vi "Dryer.vi"() -> ()   [LabVIEW 2019]
uses:
  <vilib>/NI/Current Value Table/Type Defs/Single Tag.ctl
  <vilib>/NI/Current Value Table/Type Defs/Data Types.ctl
  <vilib>/NI/STM/TCP/Read Meta Data (TCP Ref).vi
  <vilib>/NI/STM/TCP/Get Connection Reference (TCP).vi
  <vilib>/NI/AMC/Read Termination Message.vi
  <vilib>/NI/AMC/Create Single Message.vi
  <vilib>/NI/AMC/Update Message Routing Info.vi
  <vilib>/NI/STM/TCP/Read Meta Data (TCP Clst).vi
  <vilib>/NI/AMC/Globals.vi
  <vilib>/NI/STM/TCP/Write Message (TCP).vi
  <vilib>/NI/AMC/Send Message.vi
  <vilib>/NI/AMC/AMC.lvlib
  <vilib>/NI/STM/NI STM.lvlib
  <vilib>/NI/Current Value Table/Current Value Table.lvlib
panel:
  in  "Drying Flow %":dbl(knob)=5.0 min=5.0 max=50.0 step=0.1 scale=0.0..100.0
  in  "Standby Flow %":dbl(knob)=5.0 min=5.0 max=50.0 step=0.1 scale=0.0..100.0
  in  "PlenumWtrT Last Hr":bool
  out "Plenum Water Exit T":dbl(slide) scale=0.0..100.0
  in  "DryerBlrVlv Last Hr":bool
  in  "DryerT Last Hr":bool
  out "Boiler Water Valve Position":dbl(knob) scale=0.0..100.0
  out "E Stop":bool
  out "Run Enabled?":bool
  out "Actual Temperature":dbl(knob) scale=0.0..100.0
  in  "Temperature Setpoint":dbl(knob)=20.0 min=20.0 max=70.0 step=1.0 scale=20.0..70.0
  in  "Enable Dryer":bool
  in  "Machine":bool
  in  "Basement 4":bool
  in  "Dryer":bool
  in  "Rinse 4":bool
  in  "Rinse 3":bool
  in  "Rinse 2":bool
  in  "Basement 3":bool
  in  "Basement 2":bool
  in  "Basement 1":bool
  in  "Plater 6":bool
  in  "Plater 5":bool
  in  "Plater 4":bool
  in  "Plater 3":bool
  in  "Plater 2":bool
  in  "Plater 1":bool
  in  "Predip":bool
  in  "Rinse 1":bool
  in  "Cleaner":bool
  in  "Etch":bool
  out "status":string
  # "Module Selection"
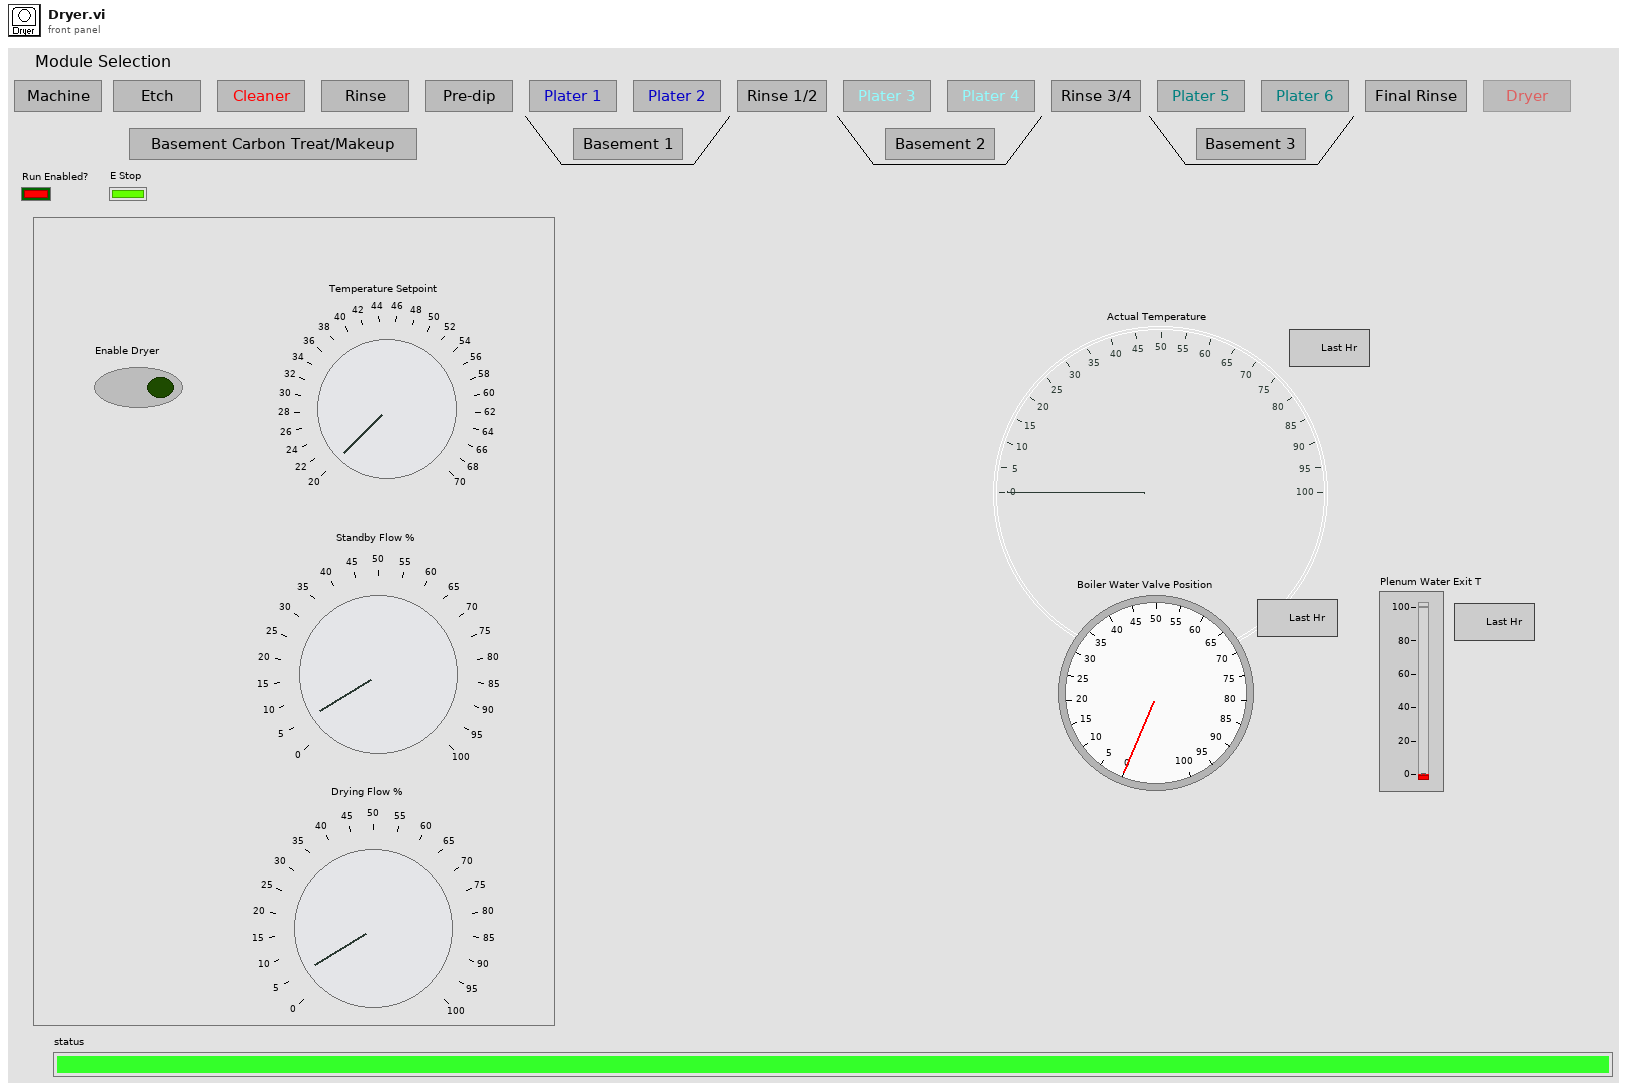
[diagram p1: front panel]
types:
  T1 = typedef "Current Value Table.lvlib/Single Tag.ctl" = cluster{"Data Type":T2, "Name":string, "Value":string, "Description":string}
  T2 = typedef "Current Value Table.lvlib/Data Types.ctl" = enum16{"Double", "Single", "I64", "I32", "I16", "I8", "U64", "U32", "U16", "U8", "String", "Boolean", "Array of U8", "Array of U16", "Array of U32", "Array of U64", "Array of I64", "Array of I32", "Array of I16", "Array of I8", "Array of Double", "Array of Single", "Array of Boolean", "Array of String"}
  T3 = typedef "NI STM.lvlib/TCP Connection Info.ctl" = cluster{"connection ID":refnum<k5>, "meta data":T4[]}
  T4 = typedef "NI STM.lvlib/MetaDataElement.ctl" = string
  T5 = typedef "AMC.lvlib/Message Queue.ctl" = refnum<queue>
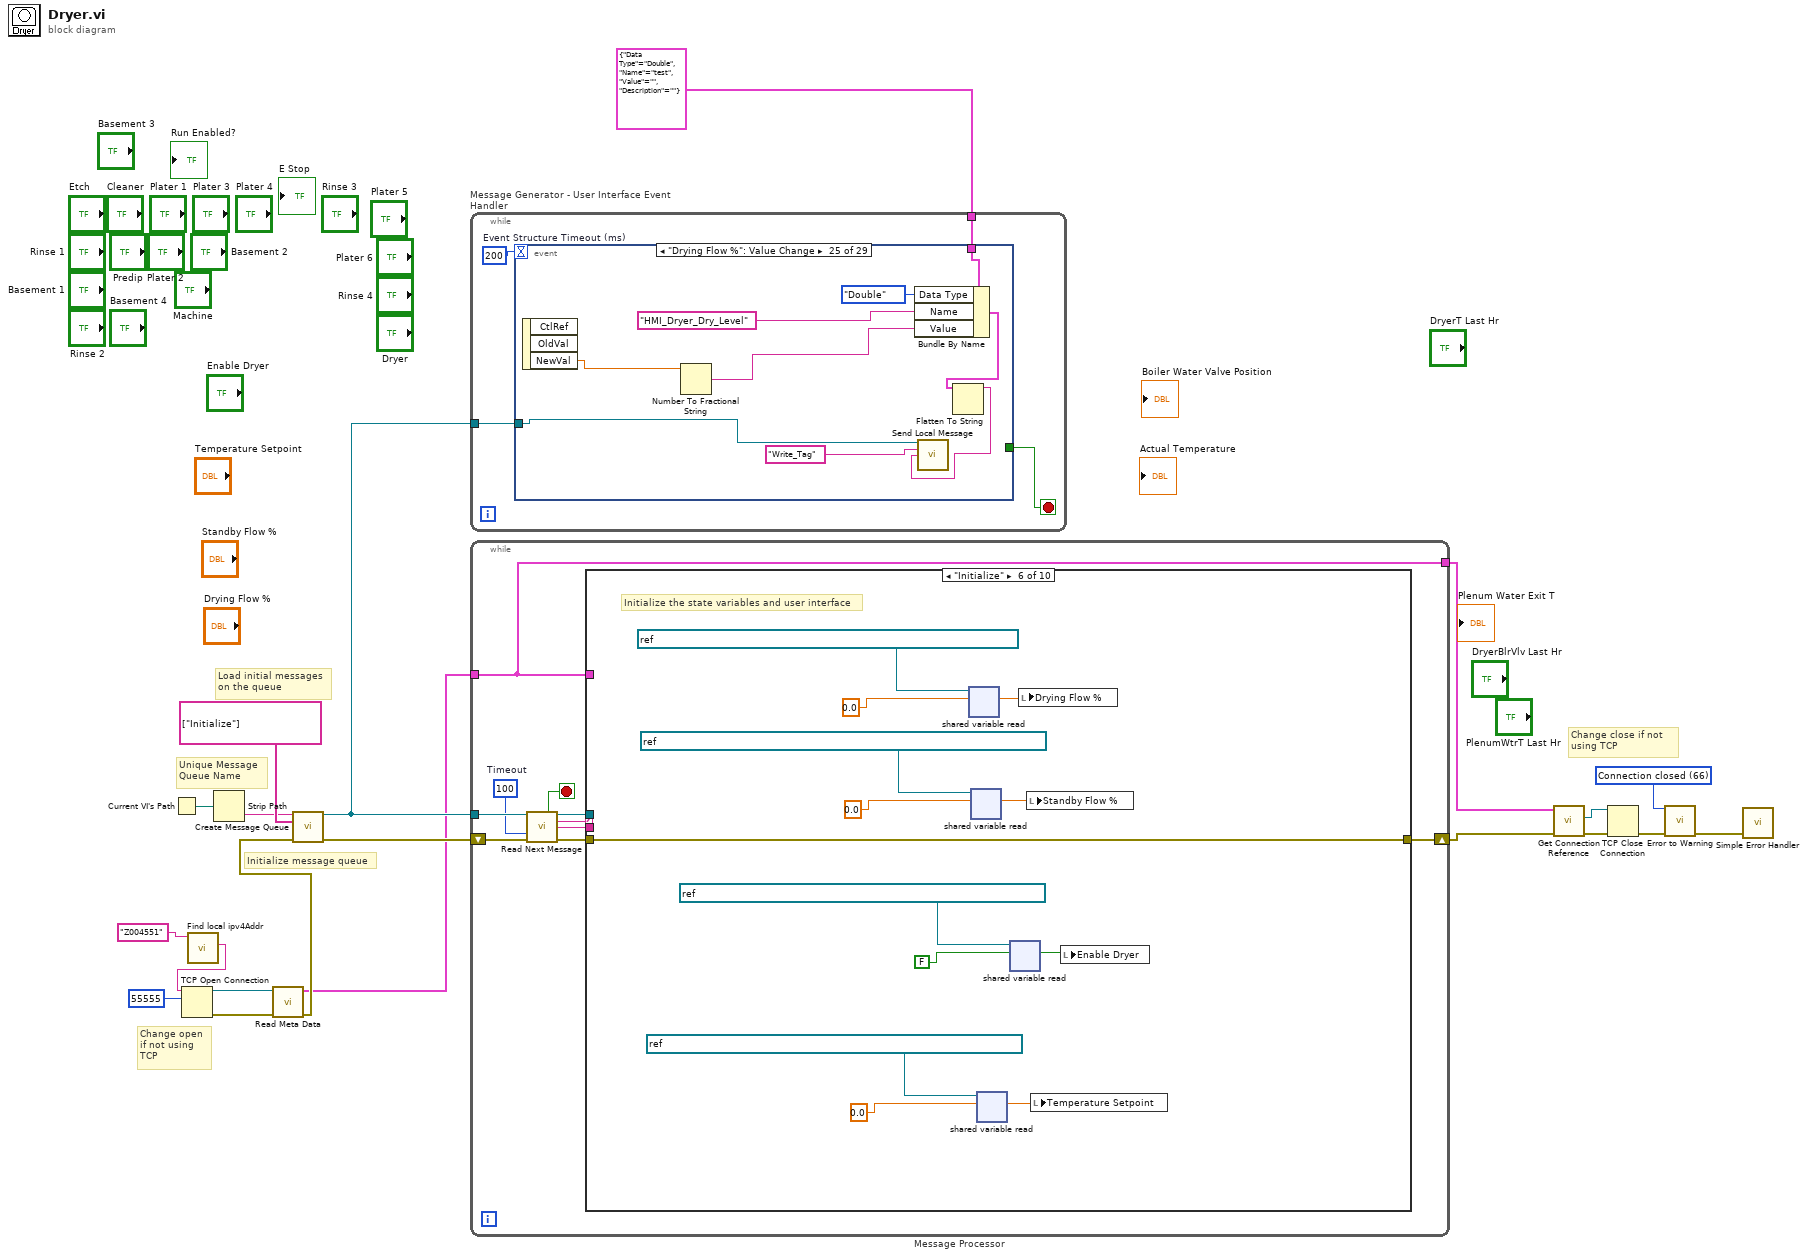
[diagram p0: block diagram]
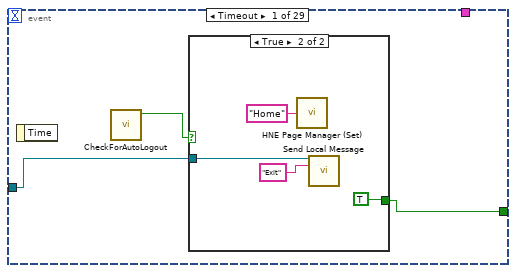
[diagram p2: hidden frame]
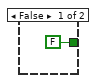
[diagram p3: hidden frame]
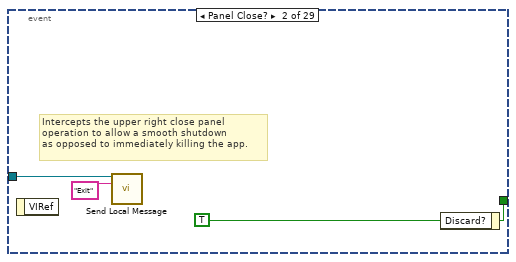
[diagram p4: hidden frame]
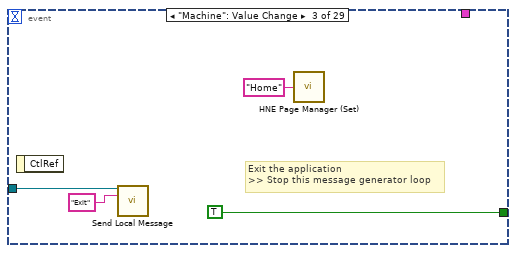
[diagram p5: hidden frame]
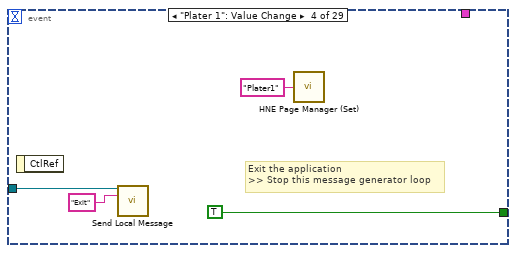
[diagram p6: hidden frame]
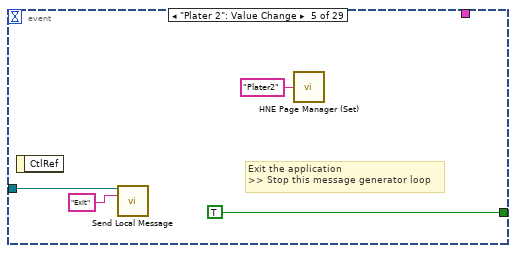
[diagram p7: hidden frame]
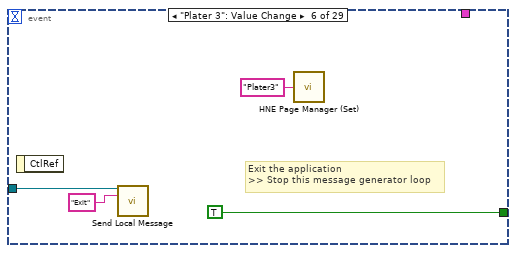
[diagram p8: hidden frame]
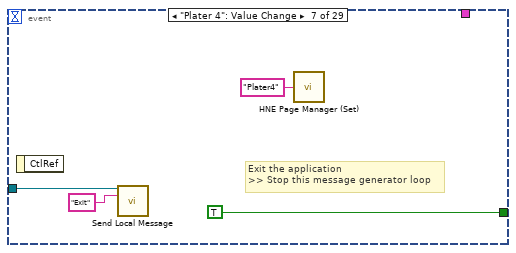
[diagram p9: hidden frame]
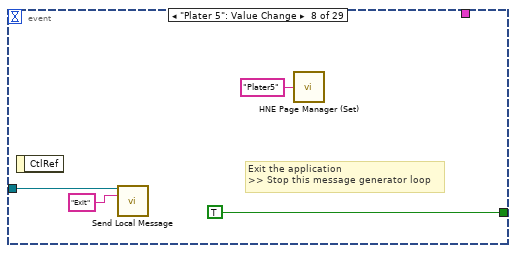
[diagram p10: hidden frame]
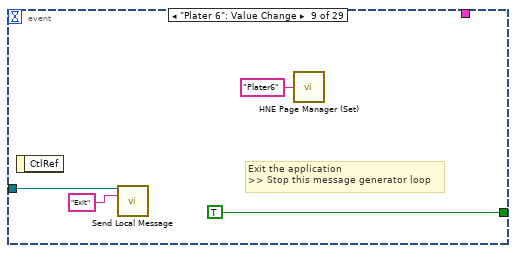
[diagram p11: hidden frame]
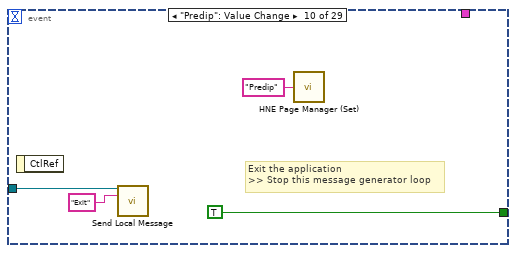
[diagram p12: hidden frame]
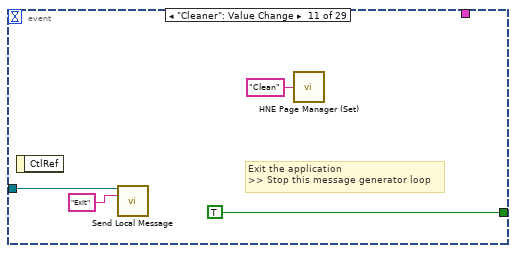
[diagram p13: hidden frame]
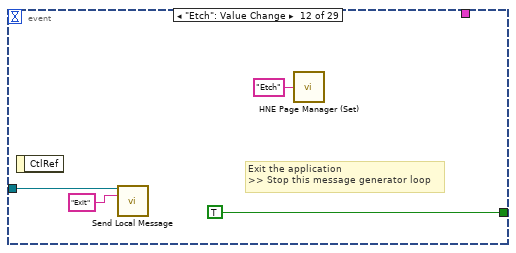
[diagram p14: hidden frame]
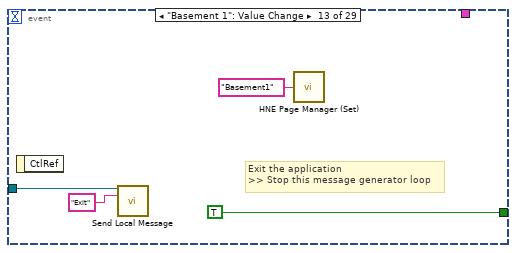
[diagram p15: hidden frame]
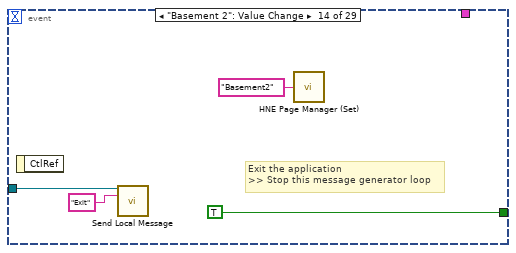
[diagram p16: hidden frame]
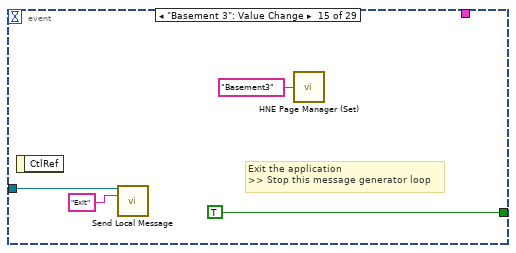
[diagram p17: hidden frame]
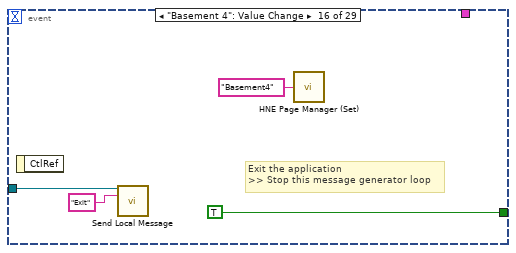
[diagram p18: hidden frame]
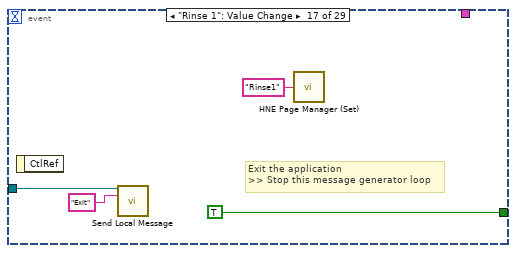
[diagram p19: hidden frame]
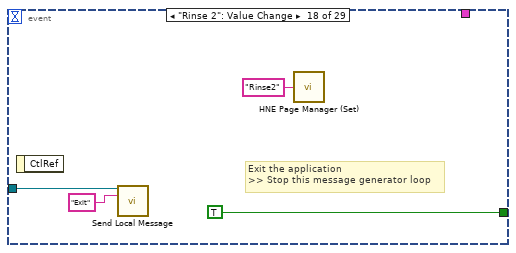
[diagram p20: hidden frame]
diagram:
  w9 = 66 items=["No Error", "Argument Error", "Memory Full", "Out of Zone", "End of File", "File Already Open", "Generic File IO Error", "File Not Found", "File Permission Error", "Disk Full", "Duplicate Path", "Too Many Files Open", "Not Enabled", "Resource File Not Found", "Cannot Add Resource", "Resource Not Found", "Image Not Found", "Image Memory Error", "Pen Does Not Exist", "Config Bad Type", "Config Token Not Found", "Config Parse Error", "Config Memory Error", "Bad External Code Format", "Bad External Code Offset", "External Code Not Present", "Null Window", "Destroy Window Mixup", "Null Menu", "Print Aborted", "Bad Print Record", "Print Driver Error", "Windows Error During Print", "Memory Error During Print", "Print Dialog Error", "Generic Print Error", "Invalid Device Refnum", "Device Not Found", "Device Parameter Error", "Device Unit Error", "Can't Open Device", "Device Call Aborted", "Generic Error", "Cancelled By User", "Object ID Too Low", "Object ID Too High", "Object Not In Heap", "Unknown Heap", "Bad DefProc ID", "DefProc Not In Table", "Message Out Of Range", "Null Method", "Unknown Message", "Manager Call Not Supported", "Bad address", "Connection In progress", "Connection timed out", "Connection is already in progress", "Network attribute not supported", "Network error", "Address in use", "System out of memory", "Connection aborted", "Connection refused", "Connection is not connected", "Connection is already connected", "Connection closed", "Initialize error (interapplication manager)", "Bad occurrence", "Wait on unbound occurrence handler", "Occurrence queue overflow", "Bad path", "Semaphore not signaled", "Unrecognized type (interapplication manager)"] ("1st Error to Convert")
  # "Change close if not using TCP"
  # "Change open if not using TCP"
  # "Initialize message queue"
  # "Unique Message\nQueue Name"
  # "Load initial messages\non the queue"
  n1 = Current VI's Path() -> (path=w16:path)
  n2 = call "Find local ipv4Addr.vi"("MachineToFind"="Z004551" ("Target IP Address")) -> ("name"=w2:string)  [unwired: 9 in, 1 out]
  n3 = TCP Open Connection(address=w2, remote port or service name=u16 55555 ("remote port")) -> (connection ID=w14:refnum<k5>, error out=w13:errorcluster)  [unwired: 1 in, 2 out]
  n4 = Strip Path(path=w16) -> (name=w19:string)  [unwired: 1 out]
  n5 = call-poly <vilib>:"Read Meta Data.vi"("error in"=w13, "connection ID"=w14) -> ("error out"=w12:errorcluster, "connection info out"=w11:T3)  [unwired: 7 in, 1 out]
  n6 = call <vilib>:"Create Message Queue.vi"("message queue name"=w19, "initial message names"=string[] ["Initialize"], "error in"=w12) -> ("message queue out"=w18:T5, "error out"=w17:errorcluster)  [unwired: 11 in]
  n7 = while "Message Generator - User Interface Event Handler" {
    tunnel: w18 -> [w22]
    tunnel: T1 {"Data Type"=enum."Double", "Name"="test", "Value"="", "Description"=""} ("Tag") -> [w21]
    stop <- w23 stop-if-true
    w24 = 200  # Event Structure Timeout (ms)
    n8 = event shown="[24] \"Drying Flow %\": Value Change" {
      selector: _ -> [_ _ _ _ _ _ _ _ _ _ _ _ _ _ _ _ _ _ _ _ _ _ _ _ _ _ _ _ _]
      dyn-events: _ -> [_ _ _ _ _ _ _ _ _ _ _ _ _ _ _ _ _ _ _ _ _ _ _ _ _ _ _ _ _]
      timeout: w24 -> [_ _ _ _ _ _ _ _ _ _ _ _ _ _ _ _ _ _ _ _ _ _ _ _ _ _ _ _ _]
      tunnel: [w25 w35 TRUE ("Discard?") TRUE ("Discard?") TRUE ("Discard?") TRUE ("Discard?") TRUE ("Discard?") TRUE ("Discard?") TRUE ("Discard?") TRUE ("Discard?") TRUE ("Discard?") TRUE ("Discard?") TRUE ("Discard?") TRUE ("Discard?") TRUE ("Discard?") TRUE ("Discard?") TRUE ("Discard?") TRUE ("Discard?") TRUE ("Discard?") TRUE ("Discard?") TRUE ("Discard?") _ _ _ _ _ _ _ _] -> w23
      tunnel: w22 -> [w26 w33 w37 w41 w45 w49 w53 w57 w61 w65 w69 w73 w77 w81 w85 w89 w93 w97 w101 w105 w109 w115 w126 w135 w144 w149 w154 w159 w164]
      tunnel: w21 -> [_ _ _ _ _ _ _ _ _ _ _ _ _ _ _ _ _ _ _ _ _ w113 w125 w134 w143 _ _ _ _]
      event Timeout {
        n9 = event-data() -> ()  [unwired: 2 out]
        n10 = call "CheckForAutoLogout.vi"() -> ("Boolean"=w27:bool)  [unwired: 11 in]
        n11 = case shown="True" w27 {
          tunnel: [FALSE ("Discard?") TRUE ("Discard?")] -> w25
          tunnel: w26 -> [_ w29]
          frame False {
          }
          frame True {
            n12 = call <userlib>:"HNE Page Manager (Set).vi"("Next Page"="Home") -> ()  [unwired: 4 in, 1 out]
            n13 = call <vilib>:"Send Local Message.vi"("message queue in"=w29, "message name"="Exit") -> ()  [unwired: 11 in, 3 out]
          }
        }
      }
      event Panel Close? {
        w35 = TRUE ("Discard?")
        # "Intercepts the upper right close panel\noperation to allow a smooth shutdown\nas opposed to immediately killing the app."
        n14 = event-data() -> ()  [unwired: 2 out]
        n15 = call <vilib>:"Send Local Message.vi"("message queue in"=w33, "message name"="Exit") -> ()  [unwired: 11 in, 3 out]
        n16 = event-data("Discard?"=w35) -> ()  [unwired: 1 in, 1 out]
      }
      event "Machine": Value Change {
        # "Exit the application\n>> Stop this message generator loop"
        n17 = event-data() -> ()  [unwired: 2 out]
        n18 = call <vilib>:"Send Local Message.vi"("message queue in"=w37, "message name"="Exit") -> ()  [unwired: 11 in, 3 out]
        n19 = call <userlib>:"HNE Page Manager (Set).vi"("Next Page"="Home") -> ()  [unwired: 4 in, 1 out]
      }
      event "Plater 1": Value Change {
        # "Exit the application\n>> Stop this message generator loop"
        n20 = event-data() -> ()  [unwired: 2 out]
        n21 = call <vilib>:"Send Local Message.vi"("message queue in"=w41, "message name"="Exit") -> ()  [unwired: 11 in, 3 out]
        n22 = call <userlib>:"HNE Page Manager (Set).vi"("Next Page"="Plater1") -> ()  [unwired: 4 in, 1 out]
      }
      event "Plater 2": Value Change {
        # "Exit the application\n>> Stop this message generator loop"
        n23 = event-data() -> ()  [unwired: 2 out]
        n24 = call <vilib>:"Send Local Message.vi"("message queue in"=w45, "message name"="Exit") -> ()  [unwired: 11 in, 3 out]
        n25 = call <userlib>:"HNE Page Manager (Set).vi"("Next Page"="Plater2") -> ()  [unwired: 4 in, 1 out]
      }
      event "Plater 3": Value Change {
        # "Exit the application\n>> Stop this message generator loop"
        n26 = event-data() -> ()  [unwired: 2 out]
        n27 = call <vilib>:"Send Local Message.vi"("message queue in"=w49, "message name"="Exit") -> ()  [unwired: 11 in, 3 out]
        n28 = call <userlib>:"HNE Page Manager (Set).vi"("Next Page"="Plater3") -> ()  [unwired: 4 in, 1 out]
      }
      event "Plater 4": Value Change {
        # "Exit the application\n>> Stop this message generator loop"
        n29 = event-data() -> ()  [unwired: 2 out]
        n30 = call <vilib>:"Send Local Message.vi"("message queue in"=w53, "message name"="Exit") -> ()  [unwired: 11 in, 3 out]
        n31 = call <userlib>:"HNE Page Manager (Set).vi"("Next Page"="Plater4") -> ()  [unwired: 4 in, 1 out]
      }
      event "Plater 5": Value Change {
        # "Exit the application\n>> Stop this message generator loop"
        n32 = event-data() -> ()  [unwired: 2 out]
        n33 = call <vilib>:"Send Local Message.vi"("message queue in"=w57, "message name"="Exit") -> ()  [unwired: 11 in, 3 out]
        n34 = call <userlib>:"HNE Page Manager (Set).vi"("Next Page"="Plater5") -> ()  [unwired: 4 in, 1 out]
      }
      event "Plater 6": Value Change {
        # "Exit the application\n>> Stop this message generator loop"
        n35 = event-data() -> ()  [unwired: 2 out]
        n36 = call <vilib>:"Send Local Message.vi"("message queue in"=w61, "message name"="Exit") -> ()  [unwired: 11 in, 3 out]
        n37 = call <userlib>:"HNE Page Manager (Set).vi"("Next Page"="Plater6") -> ()  [unwired: 4 in, 1 out]
      }
      event "Predip": Value Change {
        # "Exit the application\n>> Stop this message generator loop"
        n38 = event-data() -> ()  [unwired: 2 out]
        n39 = call <vilib>:"Send Local Message.vi"("message queue in"=w65, "message name"="Exit") -> ()  [unwired: 11 in, 3 out]
        n40 = call <userlib>:"HNE Page Manager (Set).vi"("Next Page"="Predip") -> ()  [unwired: 4 in, 1 out]
      }
      event "Cleaner": Value Change {
        # "Exit the application\n>> Stop this message generator loop"
        n41 = event-data() -> ()  [unwired: 2 out]
        n42 = call <vilib>:"Send Local Message.vi"("message queue in"=w69, "message name"="Exit") -> ()  [unwired: 11 in, 3 out]
        n43 = call <userlib>:"HNE Page Manager (Set).vi"("Next Page"="Clean") -> ()  [unwired: 4 in, 1 out]
      }
      event "Etch": Value Change {
        # "Exit the application\n>> Stop this message generator loop"
        n44 = event-data() -> ()  [unwired: 2 out]
        n45 = call <vilib>:"Send Local Message.vi"("message queue in"=w73, "message name"="Exit") -> ()  [unwired: 11 in, 3 out]
        n46 = call <userlib>:"HNE Page Manager (Set).vi"("Next Page"="Etch") -> ()  [unwired: 4 in, 1 out]
      }
      event "Basement 1": Value Change {
        # "Exit the application\n>> Stop this message generator loop"
        n47 = event-data() -> ()  [unwired: 2 out]
        n48 = call <vilib>:"Send Local Message.vi"("message queue in"=w77, "message name"="Exit") -> ()  [unwired: 11 in, 3 out]
        n49 = call <userlib>:"HNE Page Manager (Set).vi"("Next Page"="Basement1") -> ()  [unwired: 4 in, 1 out]
      }
      event "Basement 2": Value Change {
        # "Exit the application\n>> Stop this message generator loop"
        n50 = event-data() -> ()  [unwired: 2 out]
        n51 = call <vilib>:"Send Local Message.vi"("message queue in"=w81, "message name"="Exit") -> ()  [unwired: 11 in, 3 out]
        n52 = call <userlib>:"HNE Page Manager (Set).vi"("Next Page"="Basement2") -> ()  [unwired: 4 in, 1 out]
      }
      event "Basement 3": Value Change {
        # "Exit the application\n>> Stop this message generator loop"
        n53 = event-data() -> ()  [unwired: 2 out]
        n54 = call <vilib>:"Send Local Message.vi"("message queue in"=w85, "message name"="Exit") -> ()  [unwired: 11 in, 3 out]
        n55 = call <userlib>:"HNE Page Manager (Set).vi"("Next Page"="Basement3") -> ()  [unwired: 4 in, 1 out]
      }
      event "Basement 4": Value Change {
        # "Exit the application\n>> Stop this message generator loop"
        n56 = event-data() -> ()  [unwired: 2 out]
        n57 = call <vilib>:"Send Local Message.vi"("message queue in"=w89, "message name"="Exit") -> ()  [unwired: 11 in, 3 out]
        n58 = call <userlib>:"HNE Page Manager (Set).vi"("Next Page"="Basement4") -> ()  [unwired: 4 in, 1 out]
      }
      event "Rinse 1": Value Change {
        # "Exit the application\n>> Stop this message generator loop"
        n59 = event-data() -> ()  [unwired: 2 out]
        n60 = call <vilib>:"Send Local Message.vi"("message queue in"=w93, "message name"="Exit") -> ()  [unwired: 11 in, 3 out]
        n61 = call <userlib>:"HNE Page Manager (Set).vi"("Next Page"="Rinse1") -> ()  [unwired: 4 in, 1 out]
      }
      event "Rinse 2": Value Change {
        # "Exit the application\n>> Stop this message generator loop"
        n62 = event-data() -> ()  [unwired: 2 out]
        n63 = call <vilib>:"Send Local Message.vi"("message queue in"=w97, "message name"="Exit") -> ()  [unwired: 11 in, 3 out]
        n64 = call <userlib>:"HNE Page Manager (Set).vi"("Next Page"="Rinse2") -> ()  [unwired: 4 in, 1 out]
      }
      event "Rinse 3": Value Change {
        # "Exit the application\n>> Stop this message generator loop"
        n65 = event-data() -> ()  [unwired: 2 out]
        n66 = call <vilib>:"Send Local Message.vi"("message queue in"=w101, "message name"="Exit") -> ()  [unwired: 11 in, 3 out]
        n67 = call <userlib>:"HNE Page Manager (Set).vi"("Next Page"="Rinse3") -> ()  [unwired: 4 in, 1 out]
      }
      event "Rinse 4": Value Change {
        # "Exit the application\n>> Stop this message generator loop"
        n68 = event-data() -> ()  [unwired: 2 out]
        n69 = call <vilib>:"Send Local Message.vi"("message queue in"=w105, "message name"="Exit") -> ()  [unwired: 11 in, 3 out]
        n70 = call <userlib>:"HNE Page Manager (Set).vi"("Next Page"="Rinse4") -> ()  [unwired: 4 in, 1 out]
      }
      event "Dryer": Value Change {
        # "Exit the application\n>> Stop this message generator loop"
        n71 = event-data() -> ()  [unwired: 2 out]
        n72 = call <vilib>:"Send Local Message.vi"("message queue in"=w109, "message name"="Exit") -> ()  [unwired: 11 in, 3 out]
        n73 = call <userlib>:"HNE Page Manager (Set).vi"("Next Page"="Dryer") -> ()  [unwired: 4 in, 1 out]
      }
      event "Enable Dryer": Value Change {
        n74 = event-data() -> ("NewVal"=w114:bool)  [unwired: 2 out]
        n75 = Boolean To (0,1)(Boolean=w114) -> (0, 1=w120:i16)
        n76 = Number To Decimal String(number=w120) -> (decimal integer string=w117:string)  [unwired: 1 in]
        n77 = Bundle By Name(cluster=w113, "Data Type"=Data_Types."Boolean", "Name"="HMI_Dryer_Enable", "Value"=w117) -> (w112:T1)
        n78 = Flatten To String(anything=w112) -> (data string=w116:string)  [unwired: 3 in, 2 out]
        n79 = call <vilib>:"Send Local Message.vi"("message queue in"=w115, "message name"="Write_Tag", "message value"=w116) -> ()  [unwired: 10 in, 3 out]
      }
      event "Temperature Setpoint": Value Change {
        n80 = event-data() -> ("NewVal"=w123:dbl)  [unwired: 3 out]
        n81 = Number To Fractional String(number=w123) -> (F-format string=w122:string)  [unwired: 3 in]
        n82 = Bundle By Name(cluster=w125, "Data Type"=Data_Types."Double", "Name"="HMI_Dryer_T_SetPnt", "Value"=w122) -> (w124:T1)
        n83 = Flatten To String(anything=w124) -> (data string=w127:string)  [unwired: 3 in, 2 out]
        n84 = call <vilib>:"Send Local Message.vi"("message queue in"=w126, "message name"="Write_Tag", "message value"=w127) -> ()  [unwired: 10 in, 3 out]
      }
      event "Standby Flow %": Value Change {
        n85 = event-data() -> ("NewVal"=w132:dbl)  [unwired: 3 out]
        n86 = Number To Fractional String(number=w132) -> (F-format string=w131:string)  [unwired: 3 in]
        n87 = Bundle By Name(cluster=w134, "Data Type"=Data_Types."Double", "Name"="HMI_Dryer_Standby_Level", "Value"=w131) -> (w133:T1)
        n88 = Flatten To String(anything=w133) -> (data string=w136:string)  [unwired: 3 in, 2 out]
        n89 = call <vilib>:"Send Local Message.vi"("message queue in"=w135, "message name"="Write_Tag", "message value"=w136) -> ()  [unwired: 10 in, 3 out]
      }
      event "Drying Flow %": Value Change {
        n90 = event-data() -> ("NewVal"=w141:dbl)  [unwired: 3 out]
        n91 = Number To Fractional String(number=w141) -> (F-format string=w140:string)  [unwired: 3 in]
        n92 = Bundle By Name(cluster=w143, "Data Type"=Data_Types."Double", "Name"="HMI_Dryer_Dry_Level", "Value"=w140) -> (w142:T1)
        n93 = Flatten To String(anything=w142) -> (data string=w145:string)  [unwired: 3 in, 2 out]
        n94 = call <vilib>:"Send Local Message.vi"("message queue in"=w144, "message name"="Write_Tag", "message value"=w145) -> ()  [unwired: 10 in, 3 out]
      }
      event "DryerT Last Hr": Value Change {
        n95 = event-data() -> ("NewVal"=w150:bool)  [unwired: 6 out]
        n96 = case shown="True" w150 {
          tunnel: w149 -> [_ w153]
          frame False {
          }
          frame True {
            n97 = call <vilib>:"Send Local Message.vi"("message queue in"=w153, "message name"="DisplayLastHr", "message value"="Dryer_Temperature") -> ()  [unwired: 10 in, 3 out]
          }
        }
      }
      event "DryerBlrVlv Last Hr": Value Change {
        n98 = event-data() -> ("NewVal"=w155:bool)  [unwired: 6 out]
        n99 = case shown="True" w155 {
          tunnel: w154 -> [_ w158]
          frame False {
          }
          frame True {
            n100 = call <vilib>:"Send Local Message.vi"("message queue in"=w158, "message name"="DisplayLastHr", "message value"="Dryer_BlrWtrActl") -> ()  [unwired: 10 in, 3 out]
          }
        }
      }
      event "PlenumWtrT Last Hr": Value Change {
        n101 = event-data() -> ("NewVal"=w160:bool)  [unwired: 6 out]
        n102 = case shown="True" w160 {
          tunnel: w159 -> [_ w163]
          frame False {
          }
          frame True {
            n103 = call <vilib>:"Send Local Message.vi"("message queue in"=w163, "message name"="DisplayLastHr", "message value"="PlenumWtrExit_T") -> ()  [unwired: 10 in, 3 out]
          }
        }
      }
      event Menu Selection (User) {
        # "Add run-time menu items to the message\nqueue. The message handler case names must match the menu ItemTag names."
        n104 = event-data() -> ("ItemTag"=w165:string)  [unwired: 1 out]
        n105 = call <vilib>:"Send Local Message.vi"("message queue in"=w164, "message name"=w165) -> ()  [unwired: 11 in, 3 out]
      }
    }
  }
  n106 = while "Message Processor" {
    shift-left: w17 -> [w171]
    shift-right: [w175] -> w4
    tunnel: w18 -> [w172]
    tunnel: w11 -> [w166]
    tunnel: [w166] -> w5
    stop <- w174 stop-if-true
    w167 = 100  # Timeout
    n107 = call <vilib>:"Read Next Message.vi"("message queue in"=w172, "timeout (1 ms)"=w167, "error in"=w171) -> ("exit process?"=w174:bool, "message queue out"=w173:T5, "message name"=w169:string, "message value"=w168:string, "error out"=w170:errorcluster)  [unwired: 5 in, 3 out]
    n108 = case shown="\"Initialize\"" w169 {
      selector: w169 -> [_ _ w181 _ _ _ _ _ _ _]
      tunnel: w173 -> [_ _ _ _ _ _ w200 _ _ _]
      tunnel: w170 -> [w176 w178 w182 w183 w185 w198 w201 w203 w207 w209]
      tunnel: [w176 w178 w182 errorcluster {"status"=FALSE, "code"=0, "source"=""} ("error out") w185 w198 w199 w203 w206 w209] -> w175
      tunnel: w168 -> [_ _ _ _ _ _ _ _ w204 w210]
      tunnel: w166 -> [_ _ _ _ _ _ _ _ w205 _]
      frame "---------- Framework Operations ----------" {
        # "Dummy case to add a seperator in the Case Structure menu"
      }
      frame "", "Idle" {
        # "Idle Case - this case is called after a Timeout on the Get Next Message from Queue VI, if no new messages are present on the queue. This case can be used for housekeeping tasks such as updating the UI."
        n109 = control-ref of="status"() -> (w177:refnum<vi>)
        n110 = call <userlib>:"TAE Format Alarm Ticker.vi"("Alarm Ticker Ref"=w177) -> ()  [unwired: 15 in]
      }
      frame "Missing Message Handler", Default {
        # "Call this case if a message is received that is not handled \nby any other case. Typically this is a programming error\nas a result of a typo or unhandled message/missing message handler."
        n111 = Format Into String(format string="DevError: Missing message handler for '%s\" message." ("message"), w181) -> (resulting string=w179:string)  [unwired: 2 in, 1 out]
        n112 = One Button Dialog(message=w179) -> ()  [unwired: 2 out]
      }
      frame "Error" {
        # "General Error Case - this case is called if an error is passed using the error cluster below. Typically most new errors should be handed in each individual case and not passed in the rror cluster. If necessary a custom error handler case should be added and called from other cases."
        n113 = call <vilib>:"Simple Error Handler.vi"("error in (no error)"=w183) -> ()  [unwired: 1 in, 8 out]
      }
      frame "---------- Generic Operations ----------" {
        # "Dummy case to add a seperator in the Case Structure menu"
      }
      frame "Initialize" {
        # "Initialize the state variables and user interface"
        n114 = shared-variable-read(refnum<k21> "ni.var.psp://z004551/CDL0100 ReadWriteTags/HMI_Dryer_Dry_Level" ("shared variable refnum in"), 0.0) -> (w187:dbl)  [unwired: 1 in, 3 out]
        n115 = shared-variable-read(refnum<k21> "ni.var.psp://z004551/CDL0100 ReadWriteTags/HMI_Dryer_Standby_Level" ("shared variable refnum in"), 0.0) -> (w186:dbl)  [unwired: 1 in, 3 out]
        n116 = shared-variable-read(refnum<k21> "ni.var.psp://z004551/CDL0100 ReadWriteTags/HMI_Dryer_T_SetPnt" ("shared variable refnum in"), 0.0) -> (w192:dbl)  [unwired: 1 in, 3 out]
        n117 = shared-variable-read(refnum<k21> "ni.var.psp://z004551/CDL0100 ReadWriteTags/HMI_Dryer_Enable" ("shared variable refnum in"), FALSE) -> (w195:bool)  [unwired: 1 in, 3 out]
        n118 = local write "Drying Flow %"(w187) -> ()
        n119 = local write "Standby Flow %"(w186) -> ()
        n120 = local write "Temperature Setpoint"(w192) -> ()
        n121 = local write "Enable Dryer"(w195) -> ()
      }
      frame "Exit" {
        # "Destroy message queue >> this will halt the UI event handler loop"
        # "Stop the VI\n>> Perform any cleanup tasks in this message case.\n>> Clear display before closing."
        n122 = call <vilib>:"Destroy Message Queue.vi"("message queue in"=w200, "error in"=w201) -> ("error out"=w199:errorcluster)  [unwired: 11 in, 2 out]
        n123 = local write "status"("" ("Status")) -> ()
      }
      frame "---------- Application Operations ----------" {
        # "Dummy case to add a seperator in the Case Structure menu"
      }
      frame "Write_Tag" {
        n124 = call-poly <vilib>:"Write Message.vi"("error in"=w207, "data"=w204, "name"="WriteTag", "connection info in"=w205) -> ("error out"=w206:errorcluster)  [unwired: 6 in, 1 out]
      }
      frame "DisplayLastHr" {
        n125 = call "Trace Variable 1 hour Popup.vi"("Tag"=w210) -> ()  [unwired: 11 in]
      }
    }
  }
  n126 = call-poly <vilib>:"Get Connection Reference.vi"("error in"=w4, "connection info in"=w5) -> ("error out"=w8:errorcluster, "connection ID out"=w7:refnum<k5>)  [unwired: 8 out]
  n127 = TCP Close Connection(connection ID=w7, error in (no error)=w8) -> (error out=w10:errorcluster)  [unwired: 2 out]
  n128 = call <vilib>:"Error to Warning.vi"("1st Error to Convert"=w9, "error in"=w10) -> ("warning out"=w6:errorcluster)  [unwired: 3 in, 10 out]
  n129 = call <vilib>:"Simple Error Handler.vi"("error in (no error)"=w6) -> ()  [unwired: 4 in, 5 out]
